vi "Client Single Connection ICPDAS ET7000.vi"() -> ()   [LabVIEW 2021]
doc: "Demonstrates how to use Modbus functions to create a master communicating with a Modbus slave. It shows an interactive UI to allow users manually read and write the coils on the slave using TCP connection. Users can also change the timeout for reading operation if the network state is not good."
uses:
  Modbus_v121c/Modbus Data Unit/Modbus Data Unit.lvclass/Modbus Data Unit.ctl
  WebSockets/WebSocket/WebSocket.lvclass/WebSocket.ctl
  Modbus_v121c/Modbus Data Unit/Construct PDU.vi
  WebSockets/Timing/Calculate Timeout.vi
  WebSockets/WebSocket/Low-Level Read.vi
  WebSockets/WebSocket/Pong.vi
  WebSockets/Timing/Tick Count with Error Wires.vi
  Modbus_v121c/Utility/Bytes to U16s.vi
  Modbus_v121c/Master Function Definition/Function code mismatch error.vi
  Modbus_v121c/Data Model/Error Generator.vi
  Modbus_v121c/Modbus Data Unit/Deconstruct PDU.vi
  WebSockets/WebSocket/Socket Read.vi
  WebSockets/WebSocket/Low-Level Write.vi
  WebSockets/WebSocket/DataLengthBytes.vi
  WebSockets/WebSocket/EncodeMaskedBytes.vi
  WebSockets/WebSocket/Socket Write.vi
  WebSockets/WebSocket Client/WebSocket Client.lvclass
  D:/my_projects/projects/21/WebSockets/Source/WebSockets/WebSocket/WebSocket.lvclass
  <vilib>/Utility/error.llb/Error Cluster From Error Code.vi
  WebSockets/WebSocket/DecodeMaskedBytes.vi
  Modbus_v121c/Modbus Data Unit/Modbus Data Unit.lvclass
  Sockets/Socket/Socket.lvclass
  WebSockets/WebSocket/WebSocket.lvclass
  <vilib>/addons/Tools/Unicode/UTF8 Tools.lvlib
  Modbus_v121c/Master Function Definition/Master Function Definition.lvclass
  Inputs/Inputs.lvlib
panel:
  in  "write period 2":u32=500
  out "appended array":u16[](array[numeric]) format="%x"
  out "register values":u16[](array[numeric]) format="%x"
  out "error out":errorcluster
  in  "number of holding registers":u16=10 format="%x"
  in  "error in (no error)":errorcluster
  in  "starting address":u16 format="%x"
  in  "write period":u32=500
  in  "Data":string
  out "Chart":T1(graph)
  out "Received Data":string
  out "HTTP Headers":variant
  in  "WebSockets URL":string="ws://192.168.0.11:502"
  out "timer":u32(graph)
  in  "Stop":bool
  in  "Read":bool
  in  "Write":bool
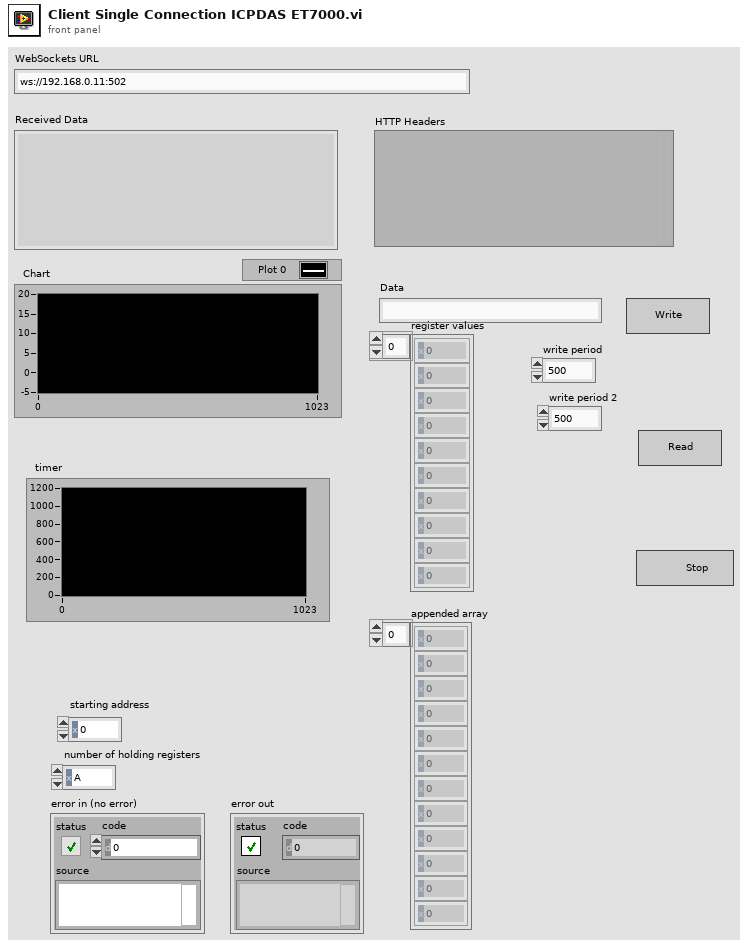
[diagram p1: front panel]
types:
  T1 = cluster{"[0]":dbl, "[1]":dbl, "[2]":dbl, "[3]":dbl, "[4]":dbl, "[5]":dbl, "[6]":dbl, "[7]":dbl, "[8]":dbl, "[9]":dbl}
  T2 = typedef "WebSockets.lvlib/WebSocket.lvclass/Opcodes.ctl" = u8
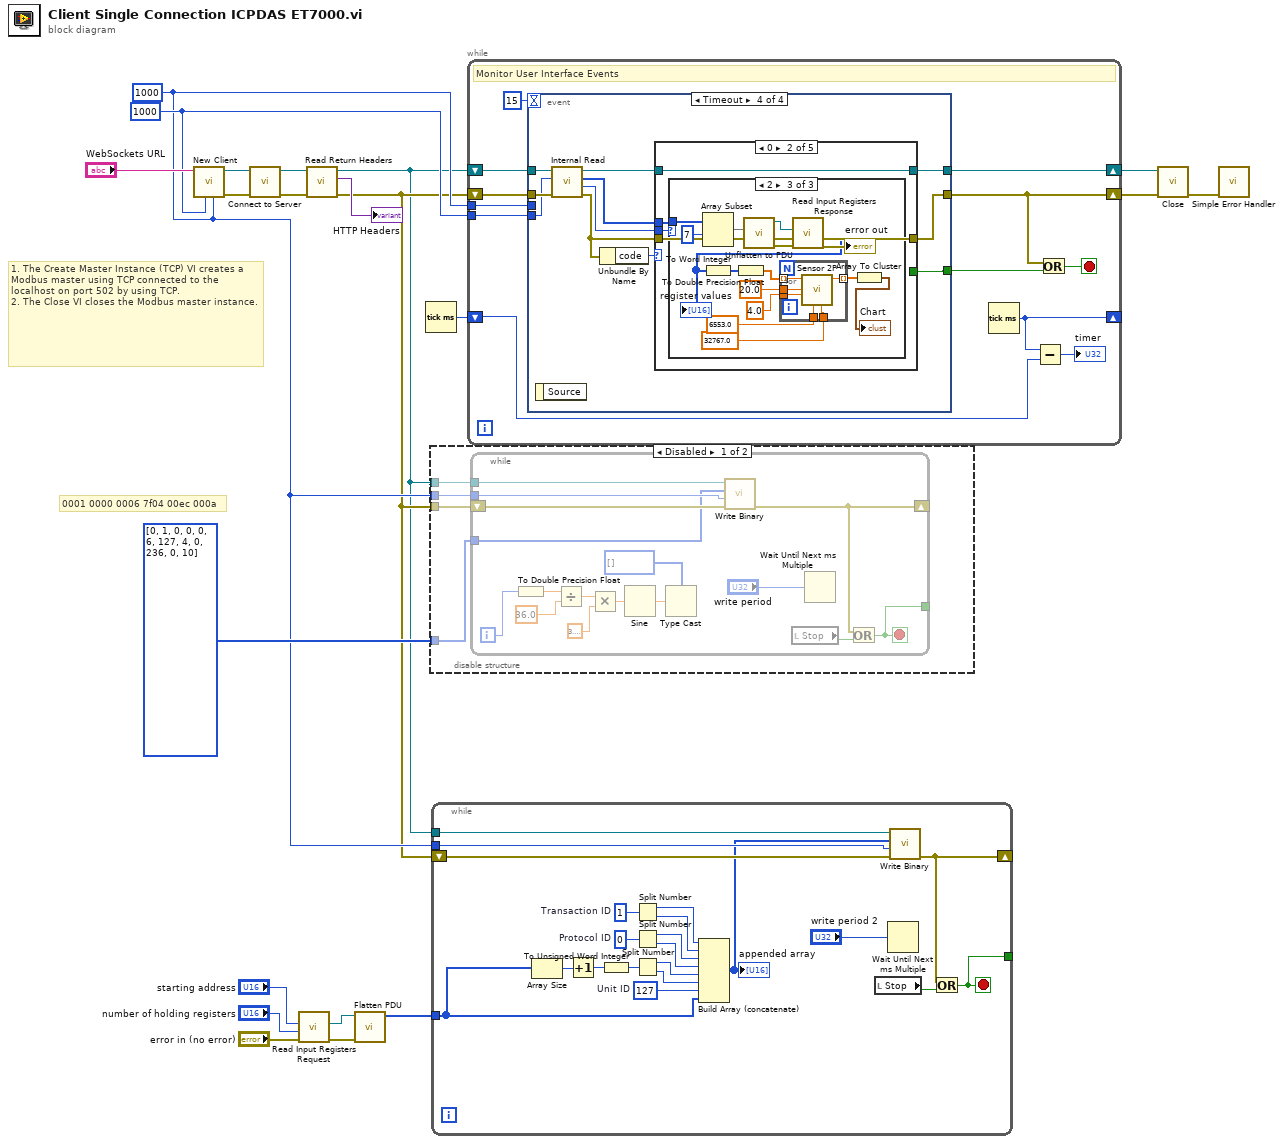
[diagram p0: block diagram]
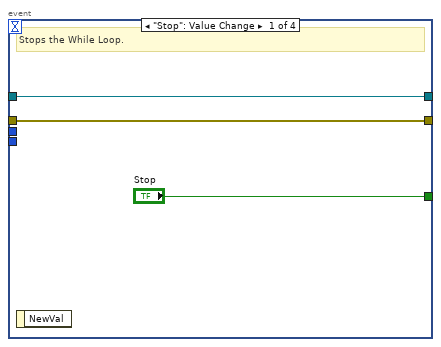
[diagram p3: hidden frame]
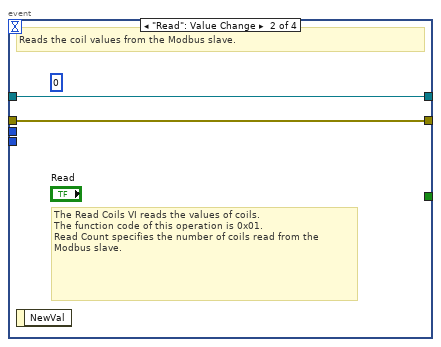
[diagram p4: hidden frame]
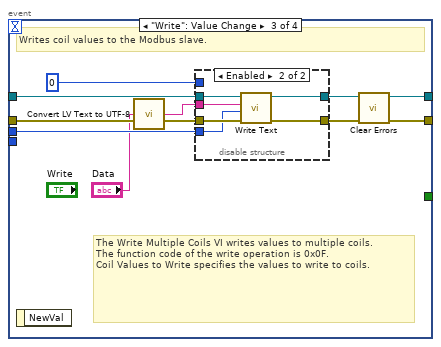
[diagram p5: hidden frame]
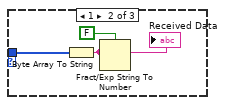
[diagram p9: hidden frame]
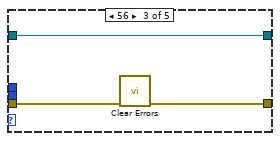
[diagram p10: hidden frame]
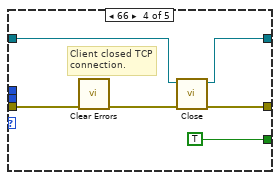
[diagram p11: hidden frame]
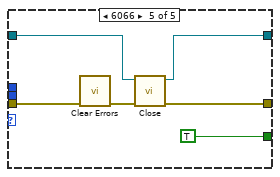
[diagram p12: hidden frame]
diagram:
  w13 = 1000 ("write operation timeout")
  w4 = 1000 ("read operation timeout")
  # "0001 0000 0006 7f04 00ec 000a"
  # "1. The Create Master Instance (TCP) VI creates a Modbus master using TCP connected to the localhost on port 502 by using TCP.\n2. The Close VI closes the Modbus master instance."
  n1 = call "New Client.vi"("write operation timeout"=w4, "read operation timeout"=w13, "WebSocket URL"="WebSockets URL") -> ("error out"=w15:errorcluster, "WebSocket Client out"=w16:refnum<class "WebSocket Client.lvclass">)  [unwired: 7 in]
  n2 = call "Connect to Server.vi"("error in (no error)"=w15, "WebSocket Client in"=w16) -> ("error out"=w11:errorcluster, "WebSocket Client out"=w12:refnum<class "WebSocket Client.lvclass">)  [unwired: 8 in]
  n3 = call "Read Input Registers Request.vi"("error in"="error in (no error)", "Number of Registers"="number of holding registers", "Starting Address"="starting address") -> ("error out"=w5:errorcluster, "modbus data unit out"=w6:refnum<class "Modbus Data Unit.lvclass">)  [unwired: 7 in]
  n4 = call "Read Return Headers.vi"("error in (no error)"=w11, "WebSocket in"=w12) -> ("error out"=w3:errorcluster, "Return Headers"=→"HTTP Headers":variant, "WebSocket out"=w2:refnum<class "WebSocket Client.lvclass">)  [unwired: 7 in]
  n5 = call "Flatten PDU.vi"("error in"=w5, "modbus data unit in"=w6) -> ("Full modbus data unit"=w1:u8[])  [unwired: 8 in, 1 out]
  n6 = Tick Count (ms)() -> (millisecond timer value=w21:u32)
  n7 = disable-structure shown="Disabled" {
    disable-tunnel: w2 -> [w25 _]
    disable-tunnel: w3 -> [w24 _]
    disable-tunnel: w4 -> [w23 _]
    disable-tunnel: u8[] [0, 1, 0, 0, 0, 6, 127, 4, 0, 236, 0, 10] ("values") -> [w22 _]
    frame Disabled {
      n8 = while {
        tunnel: w25 -> [w30]
        tunnel: [w40] -> _
        shift-right: [w29] -> _
        shift-left: w24 -> [w28]
        tunnel: w23 -> [w27]
        tunnel: w22 -> [w26]
        i -> [w31]
        stop <- w40 stop-if-true
        n9 = To Double Precision Float(number=w31) -> (double precision float=w38:dbl)
        n10 = Divide(x=w38, y=36.0) -> (x/y=w37:dbl)
        n11 = Multiply(x=w37, y=3.141592653589793) -> (x*y=w36:dbl)
        n12 = Sine(x=w36) -> (sin(x)=w35:dbl)
        n13 = Type Cast(type=u8[] [] ("values"), x=w35) -> ()  [unwired: 1 out]
        n14 = call-dynamic "Write Binary.vi"("error in (no error)"=w28, "timeout ms (5000)"=w27, "Binary Data"=w26, "WebSocket in"=w30) -> ("error out"=w29:errorcluster)  [unwired: 6 in, 1 out]
        n15 = local read "Stop"() -> (w41:bool)
        n16 = Wait Until Next ms Multiple(millisecond multiple="write period") -> ()  [unwired: 1 out]
        n17 = Or(x=w29, y=w41) -> (x .or. y?=w40:bool)
      }
    }
    frame Enabled {
    }
  }
  n18 = while {
    tunnel: w2 -> [w59]
    tunnel: [w61] -> _
    shift-right: [w58] -> _
    shift-left: w3 -> [w57]
    tunnel: w4 -> [w56]
    tunnel: w1 -> [w45]
    stop <- w61 stop-if-true
    w46 = u16 127  # Unit ID
    w44 = u32 0  # Protocol ID
    w43 = u16 1  # Transaction ID
    n19 = Array Size(array=w45) -> (size(s)=w47:i32)
    n20 = Increment(x=w47) -> (x+1=w48:i32)
    n21 = To Unsigned Word Integer(number=w48) -> (unsigned 16bit integer=w49:u16)
    n22 = Split Number(x=w43) -> (hi(x)=w50:u8, lo(x)=w51:u8)
    n23 = Split Number(x=w44) -> (hi(x)=w52:u16, lo(x)=w53:u16)
    n24 = Split Number(x=w49) -> (hi(x)=w54:u8, lo(x)=w55:u8)
    n25 = Build Array (concatenate)(w50, w51, w52, w53, w54, w55, w46, w45) -> (w42:u16[])
    "appended array" <- w42
    n26 = local read "Stop"() -> (w62:bool)
    n27 = Wait Until Next ms Multiple(millisecond multiple="write period 2") -> ()  [unwired: 1 out]
    n28 = call-dynamic "Write Binary.vi"("error in (no error)"=w57, "timeout ms (5000)"=w56, "Binary Data"=w42, "WebSocket in"=w59) -> ("error out"=w58:errorcluster)  [unwired: 6 in, 1 out]
    n29 = Or(x=w58, y=w62) -> (x .or. y?=w61:bool)
  }
  n30 = while {
    shift-right: [w73] -> w19
    shift-left: w2 -> [w74]
    shift-right: [w71] -> w18
    shift-left: w3 -> [w72]
    shift-right: [w66] -> _
    shift-left: w21 -> [w67]
    tunnel: w4 -> [w64]
    tunnel: w13 -> [w63]
    stop <- w69 stop-if-true
    # "Monitor User Interface Events"
    n31 = event shown="[3] Timeout" {
      selector: _ -> [_ _ _ _]
      dyn-events: _ -> [_ _ _ _]
      timeout: 15 -> [_ _ _ _]
      tunnel: ["Stop" _ _ w102] -> w70
      tunnel: w74 -> [w76 w78 w88 w105]
      tunnel: [w76 w78 w87 w111] -> w73
      tunnel: w72 -> [w77 w79 w83 w104]
      tunnel: [w77 w79 w85 w112] -> w71
      tunnel: w64 -> [_ _ w86 _]
      tunnel: w63 -> [_ _ _ w103]
      event "Stop": Value Change {
        # "Stops the While Loop."
        n32 = event-data() -> ()  [unwired: 1 in, 1 out]
      }
      event "Read": Value Change {
        (unwired) u16 0 ("starting address")
        # "The Read Coils VI reads the values of coils.\nThe function code of this operation is 0x01.\nRead Count specifies the number of coils read from the Modbus slave."
        # "Reads the coil values from the Modbus slave."
        n33 = event-data() -> ()  [unwired: 1 in, 1 out]
      }
      event "Write": Value Change {
        # "The Write Multiple Coils VI writes values to multiple coils.\nThe function code of the write operation is 0x0F.\nCoil Values to Write specifies the values to write to coils."
        # "Writes coil values to the Modbus slave."
        n34 = event-data() -> ()  [unwired: 1 in, 1 out]
        n35 = call <vilib>:"Convert LV Text to UTF-8.vi"("LV Text"="Data", "error in"=w83) -> ("UTF-8 Text"=w80:string, "error out"=w82:errorcluster)  [unwired: 12 in]
        n36 = disable-structure shown="Enabled" {
          disable-tunnel: u16 0 ("starting address") -> [w95 _]
          disable-tunnel: w88 -> [w94 w101]
          disable-tunnel: [w93 w99] -> w87
          disable-tunnel: w82 -> [w92 w98]
          disable-tunnel: [w91 w100] -> w84
          disable-tunnel: w80 -> [w90 w97]
          disable-tunnel: w86 -> [_ w96]
          frame Disabled {
          }
          frame Enabled {
            n37 = call-dynamic "Write Text.vi"("error in (no error)"=w98, "timeout ms (5000)"=w96, "String Data"=w97, "WebSocket in"=w101) -> ("error out"=w100:errorcluster, "WebSocket out"=w99:refnum<class "WebSocket Client.lvclass">)  [unwired: 6 in]
          }
        }
        n38 = call <vilib>:"Clear Errors.vi"("error in (no error)"=w84) -> ("error out"=w85:errorcluster)  [unwired: 5 in, 1 out]
      }
      event Timeout {
        n39 = event-data() -> ()  [unwired: 1 in, 1 out]
        n40 = call "Internal Read.vi"("error in (no error)"=w104, "timeout ms"=w103, "WebSocket in"=w105) -> ("error out"=w107:errorcluster, "Opcode"=w106:T2, "Data"=w108:u8[], "WebSocket out"=w109:refnum<class "WebSocket Client.lvclass">)  [unwired: 5 in]
        n41 = Unbundle By Name(w107) -> ("code"=w110:i32)
        n42 = case shown="0" w110 {
          tunnel: w108 -> [_ w118 _ _ _]
          tunnel: [w114 w117 w144 w148 w154] -> w112
          tunnel: w107 -> [w114 w117 w145 w151 w156]
          tunnel: w109 -> [w113 w116 w143 w146 w157]
          tunnel: [w113 w116 w143 w147 w152] -> w111
          tunnel: w106 -> [_ w115 _ _ _]
          tunnel: [_ _ _ TRUE ("Stop") TRUE ("Stop")] -> w102
          frame Default {
          }
          frame 0 {
            n43 = case shown="2" w115 {
              tunnel: w118 -> [_ w121 w135]
              frame 0, Default {
              }
              frame 1 {
                n44 = Byte Array To String(unsigned byte array=w121) -> (string=w120:string)
                "Received Data" <- w120
                n45 = Fract/Exp String To Number(use system decimal point (T)=FALSE, string=w120) -> ()  [unwired: 2 in, 2 out]
              }
              frame 2 {
                n46 = Array Subset(array=w135, index=7) -> (w131:u8[])  [unwired: 1 in]
                n47 = call "Unflatten to PDU.vi"("modbus data unit data"=w131) -> ("error out"=w133:errorcluster, "modbus data unit out"=w132:refnum<class "Modbus Data Unit.lvclass">)  [unwired: 9 in]
                n48 = call "Read Input Registers Response.vi"("error in"=w133, "modbus data unit in"=w132) -> ("error out"=→"error out":errorcluster, "Register Values"=w122:u16[])  [unwired: 7 in, 1 out]
                "register values" <- w122
                n49 = To Word Integer(number=w122) -> (16bit integer=w130:i16[])
                n50 = To Double Precision Float(number=w130) -> (double precision float=w129:dbl[])
                n51 = for {
                  tunnel: w129 -> [w142] mode=indexing
                  tunnel: 6553.0 ("Xmin") -> [w141]
                  tunnel: 32767.0 ("Xmin") -> [w140]
                  tunnel: 4.0 ("Xmin") -> [w139]
                  tunnel: 20.0 ("Xmin") -> [w138]
                  tunnel: [w137] -> w124 mode=indexing
                  n52 = call "Sensor 2P.vi"("Xmax"=w140, "Xmin"=w141, "Ymin"=w139, "Ymax"=w138, "X"=w142) -> ("Y"=w137:dbl)  [unwired: 6 in]
                }
                n53 = Array To Cluster(array=w124) -> (cluster=→"Chart":T1)
              }
            }
          }
          frame 56 {
            n54 = call <vilib>:"Clear Errors.vi"("error in (no error)"=w145) -> ("error out"=w144:errorcluster)  [unwired: 5 in, 1 out]
          }
          frame 66 {
            # "Client closed TCP connection."
            n55 = call <vilib>:"Clear Errors.vi"("error in (no error)"=w151) -> ("error out"=w149:errorcluster)  [unwired: 5 in, 1 out]
            n56 = call-dynamic "Close.vi"("error in (no error)"=w149, "WebSocket Client in"=w146) -> ("error out"=w148:errorcluster, "WebSocket Client out"=w147:refnum<class "WebSocket Client.lvclass">)  [unwired: 8 in]
          }
          frame 6066 {
            n57 = call <vilib>:"Clear Errors.vi"("error in (no error)"=w156) -> ("error out"=w155:errorcluster)  [unwired: 5 in, 1 out]
            n58 = call-dynamic "Close.vi"("error in (no error)"=w155, "WebSocket Client in"=w157) -> ("error out"=w154:errorcluster, "WebSocket Client out"=w152:refnum<class "WebSocket Client.lvclass">)  [unwired: 8 in]
          }
        }
      }
    }
    n59 = Tick Count (ms)() -> (millisecond timer value=w66:u32)
    n60 = Subtract(x=w66, y=w67) -> (x-y=→"timer":u32)
    n61 = Or(x=w71, y=w70) -> (x .or. y?=w69:bool)
  }
  n62 = call-dynamic "Close.vi"("error in (no error)"=w18, "WebSocket Client in"=w19) -> ("error out"=w17:errorcluster)  [unwired: 8 in, 1 out]
  n63 = call <vilib>:"Simple Error Handler.vi"("error in (no error)"=w17) -> ()  [unwired: 4 in, 5 out]
